vi "DQMH System Message - Add to Run-Time Menu.vi"(9 "Module Descriptor":string, 11 "Main VI Reference":refnum<vi>) -> (1 "Payload":variant, 2 "Identifier":string="Add to Run-Time Menu", 5 "Source":T1)   [LabVIEW 2022 SP3, in "hse-dqmh.lvlib"]
doc: "Sends the modul's <b>Path</b> and <b>Module Descriptor</b> via the \"Add to Run-Time Menu\" System Message broadcast. The UI Manager inserts the module into the relevant locations in the run-time menu.\n\n____\nHAMPEL SOFTWARE ENGINEERING v3.8.0 (2023-12-18 14:41)"
uses:
  hse-dqmh.lvlib
  Controls/System Message Source.ctl
  Controls/System Message Framework Identifiers.ctl
  Controls/System Message - Add to Run-Time Menu - Argument--cluster.ctl
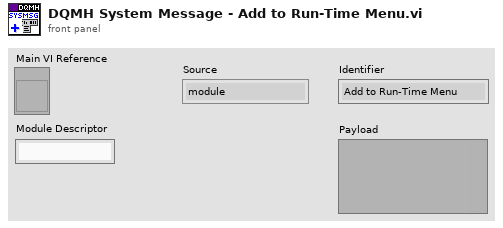
[diagram p1: front panel]
types:
  T1 = typedef "hse-dqmh.lvlib/System Message Source.ctl" = enum16{"module", "application", "network"}
  T2 = typedef "hse-dqmh.lvlib/System Message - Add to Run-Time Menu - Argument--cluster.ctl" = cluster{"Module Disk Path":path, "Module Descriptor":string}
  T3 = typedef "hse-dqmh.lvlib/System Message Framework Identifiers.ctl" = enum16{"Add to Run-Time Menu", "Ready for Display", "Removed from Subpanel", "Remove from Run-Time Menu"}
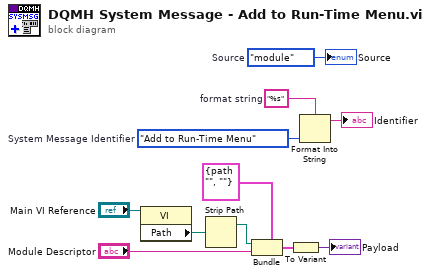
[diagram p0: block diagram]
diagram:
  w7 = "%s"  # format string
  w9 = System_Message_Framework_Identifiers."Add to Run-Time Menu"  # System Message Identifier
  w11 = System_Message_Source."module"  # Source
  n1 = property class="VI"(reference="Main VI Reference") -> ("Path"=w3:path)  [unwired: 1 in, 2 out]
  n2 = Strip Path(path=w3) -> (stripped path=w1:path)  [unwired: 1 out]
  n3 = Bundle(cluster=T2 {"Module Disk Path"=path "", "Module Descriptor"=""}, "Module Disk Path"=w1, "Module Descriptor"="Module Descriptor") -> (w5:T2)
  n4 = To Variant(anything=w5) -> (Variant=→"Payload":variant)
  n5 = Format Into String(format string=w7, w9) -> (resulting string=→"Identifier":string)  [unwired: 2 in, 1 out]
  "Source" <- w11
